vi "Local MS Auto_backup.vi"() -> ()   [LabVIEW 2016]
uses:
  Subsystems/Global Variables.vi
  <vilib>/FPGAPlugInAG/PXI-7833R/niLvFpga_Open_PXI-7833R.vi
  <vilib>/Utility/error.llb/Error Cluster From Error Code.vi
  <vilib>/rvi/errors/niLvFpgaAdjustHostInterfaceError.vi
  <vilib>/FPGAPlugInAG/PXI-7833R/niLvFpga_Reset_PXI-7833R.vi
  <vilib>/FPGAPlugInAG/PXI-7833R/niLvFpga_Close_PXI-7833R.vi
  <vilib>/rvi/interface/nirviOpenFPGA/nirviOpenFPGA.xnode
  FPGA Bitfiles/PhantomControlPI_FPGATarget_QuadCtr2_E2412E44.lvbitx
  IRISS_FPGA_IO.vi
  <vilib>/rvi/interface/nirviReadWriteControl/nirviReadWriteControl.xnode
  <vilib>/rvi/interface/nirviMethod/nirviMethod.xnode
  <vilib>/rvi/interface/nirviCloseFPGA/nirviCloseFPGA.xnode
  Library/KevinLibraryAll/labview2011/kevLib2011.lvlib
  NiFpgaLv.dll
panel:
  in  "Pause":bool caption="To M/S"
  in  "No. Cycles":u8=1
  out "Current No.":u8
  in  "L4 [deg]":dbl
  in  "L3 [mm]":dbl step=0.1
  in  "L2 [deg]":dbl
  in  "L1 [deg]":dbl
  out "Trajectory Cluster":T1
  out "Update Mdl & Traj":bool=TRUE
  out "Stage PID Cluster":T2={"Stage Z PID"={"Kp"=0.0005, "Kd"=0.001, "Ki"=0.0}, "Stage Y PID"={"Kp"=0.0003, "Kd"=0.01, "Ki"=0.0}, "Stage X PID"={"Kp"=0.0003, "Kd"=0.01, "Ki"=0.0}}
  out "L1 to L4 PID Cluster":T3={"L1 PID Gains"={"Kp"=0.005, "Kd"=0.5, "Ki"=0.0005}, "L2 PID Gains"={"Kp"=0.01, "Kd"=1.0, "Ki"=0.0005}, "L3 PID Gains"={"Kp"=0.05, "Kd"=1.0, "Ki"=0.0005}, "L4 PID Gains"={"Kp"=0.1, "Kd"=1.0, "Ki"=0.0005}}
  in  "IRISS GUI":T4(tab)
  out "X Stage out [mm] 2":dbl caption="Stage X [mm]" format="%#.4f"
  out "Z Stage out [mm] 2":dbl caption="Stage Z [mm]" format="%#.4f"
  out "Y Stage out [mm] 2":dbl caption="Stage Y [mm]" format="%#.4f"
  out "Vacuum Force [mmHg]  2":i32 caption="[mmHg]"
  out "Finished Late Counts":u16
  out "Emergency alarm":bool
  out "Remote sender engaged":bool
  in  "L2 PID Gains":cluster{"Kp":dbl, "Kd":dbl, "Ki":dbl}={"Kp"=0.01, "Kd"=1.0, "Ki"=0.005}
  in  "L3 PID Gains":cluster{"Kp":dbl, "Kd":dbl, "Ki":dbl}={"Kp"=0.05, "Kd"=1.0, "Ki"=0.0005}
  in  "L4 PID Gains":cluster{"Kp":dbl, "Kd":dbl, "Ki":dbl}={"Kp"=0.1, "Kd"=0.1, "Ki"=0.0005}
  in  "L1 PID Gains":cluster{"Kp":dbl, "Kd":dbl, "Ki":dbl}={"Kp"=0.01, "Kd"=0.5, "Ki"=0.001}
  out "Current System State":T5(ring)
  out "State changing":bool
  out "Tip out Posit":dbl[](array[numeric]) caption="Position [mm]" format="%#.3f"
  out "Tip cmd Posit":dbl[](array[numeric]) caption="Command [mm]" format="%#.3f"
  out "L4 out Posit":dbl caption="y [deg]" format="%#.2g"
  out "L4 cmd Posit":dbl caption="r [deg]" format="%#.2g"
  out "L3 out Posit":dbl caption="y [mm]" format="%#.2g"
  out "L3 cmd Posit":dbl caption="r [mm]" format="%#.2g"
  out "L2 out Posit":dbl caption="y [deg]" format="%#.2g"
  out "L2 cmd Posit":dbl caption="r [deg]" format="%#.2g"
  out "L1 out Posit":dbl caption="y [deg]" format="%#.2g"
  out "L1 cmd Posit":dbl caption="r [deg]" format="%#.2g"
  out "State Flag Array":bool[](array[boolean])
  out "Irrigation Engaged? 2":bool caption="Irrigation Engaged"
  in  "Joint Limits":dbl[][](array[numeric])=[[-8.0, 50.0], [-35.0, 35.0], [-5.0, 20.0], [-180.0, 180.0]] format="%#.3g"
  out "First Trk Pt":dbl[](array[numeric]) format="%#.3g"
  in  "Offset Home 2 RCM":dbl[](array[numeric])=[-7.7, 37.0, 55.0, 0.0] format="%#.3g"
  out "Error(s) Out on Program End":errorcluster
  out "L4 Chart":dbl(graph)
  out "L3 Chart":dbl(graph)
  out "L2 Chart":dbl(graph)
  out "L1 Chart":dbl(graph)
  in  "Clear Charts":bool
  out "AC Pressure [mmHg]":sgl
  out "Elaspsed Time":sgl
  in  "File Path":path=path "C:/KevData1.txt"
  in  "Take IOP Data":bool
  out "IOP File Exists":bool
  in  "Seconds of Data":sgl=5.0
  in  "Irrigation?":bool
  in  "PID ON/OFF":bool
  in  "Vac PID Gains":cluster{"Kp":dbl, "Kd":dbl, "Ki":dbl, "Ts":dbl}={"Kp"=5.0, "Kd"=0.0, "Ki"=5.0, "Ts"=0.01}
  in  "Vac Cmd":sgl min=0 max=100 step=1 format="%#_13g"
  in  "Target IOP":sgl=20.0 min=0 max=100 step=1 format="%#_13g"
  out "IOP Ctrl":T6(graph)
  out "Pressure Sensors":T7(graph)
  in  "Remote Control Source":u16(ring) caption="Remote Source" items=["Surgical Console", "Joystick"]
  in  "Reset Joystick":bool caption="Encoder Reset"
  in  "max limit [mmHg]":dbl=600.0
  out "OCT Z out [mm]":dbl caption="OCT Out Z [mm]" format="%#.4f"
  out "OCT Z cmd [mm]":dbl=6.0 caption="OCT Z Ref [mm]" min=0.0 max=12.0 step=0.5
  in  "OCT Z PID Gains":cluster{"Kp":dbl, "Kd":dbl, "Ki":dbl}={"Kp"=0.0003, "Kd"=0.0001, "Ki"=0.01}
  out "Z Stage out [mm]":dbl caption="Output Z [mm]" format="%#.4f"
  out "Z Stage cmd [mm]":dbl=6.0 caption="Reference Z [mm]" min=0.0 max=12.0 step=0.5
  out "Y Stage out [mm]":dbl caption="Output Y [mm]" format="%#.4f"
  out "Y Stage cmd [mm]":dbl=6.0 caption="Reference Y  [mm]" min=0.0 max=12.0 step=0.5
  out "X Stage out [mm]":dbl caption="Output X [mm]" format="%#.4f"
  out "X Stage cmd [mm]":dbl=6.0 caption="Reference X [mm]" min=0.0 max=12.0 step=0.5
  in  "Stage Z PID Gains":cluster{"Kp":dbl, "Kd":dbl, "Ki":dbl}={"Kp"=0.0005, "Kd"=0.001, "Ki"=0.0}
  in  "Stage Y PID Gains":cluster{"Kp":dbl, "Kd":dbl, "Ki":dbl}={"Kp"=0.0001, "Kd"=0.005, "Ki"=0.0}
  in  "Stage X PID Gains":cluster{"Kp":dbl, "Kd":dbl, "Ki":dbl}={"Kp"=0.0003, "Kd"=0.01, "Ki"=0.0}
  out "Irrigation Engaged?":bool
  out "Accurus Button":bool[](array[boolean]) caption="Remote Button Command"
  in  "Control: Vacuum Force":i8(slide) min=0 max=78 step=1 scale=0.0..78.0
  out "Voltage Output Ch. B":dbl(graph)
  out "Voltage Output Ch. A":dbl(graph)
  out "Accurus Engaged?":bool
  out "Vacuum Force [mmHg]":i32
  in  "Load Traj":bool caption="To M/S"
  in  "Retract":bool caption="To M/S"
  in  "Stop Accurus":bool caption="To M/S"
  in  "L3 Go Home":bool caption="To M/S"
  in  "Track":bool caption="To M/S"
  in  "Program Stop":bool
  # "Robot Status"
  # "Reserved"
  # "Tool Tip Location"
  # "L1"
  # "X\nY\nZ"
  # "X\nY\nZ"
  # "L2"
  # "Reserved"
  # "System Progress"
  # "L3"
  # "Homing finished"
  # "Reserved"
  # "M/S initialization finished"
  # "Trajecoty loading finished"
  # "Tracking initialization finished"
  # "L4"
  # "In Tracking"
  # "Notes: \n2. check state transition\n4. preview trajectory?"
  # "Vacuum"
  # "Joint Motion"
  # "Calibration"
  # "Space Deform Parameters"
  # "L1"
  # "[deg]"
  # "S"
  # "L2"
  # "[deg]"
  # "R"
  # "[deg]"
  # "L3"
  # "[mm]"
  # "T"
  # "[mm]"
  # "L4"
  # "[deg]"
  # "First Track Point"
  # "AC & PC Gap"
  # "L1"
  # "[deg]"
  # "L2"
  # "[deg]"
  # "L3"
  # "[mm]"
  # "L4"
  # "[deg]"
  # "Error Message"
  # "Tracking Joint Limits"
  # "Incision"
  # "Min."
  # "Max."
  # "L1"
  # "L1"
  # "[deg]"
  # "L2"
  # "L2"
  # "[deg]"
  # "L3"
  # "L3"
  # "[mm]"
  # "L4"
  # "L4"
  # "[deg]"
  # "Data Saving"
  # "IOP Feedback Control"
  # "XYZ Stage Control"
  # "OCT Z-Axis"
  # "Foot Pedal Buttons"
  # "Irrigation and Aspiration"
  # "Button 1"
  # "Button 2"
  # "Button 3"
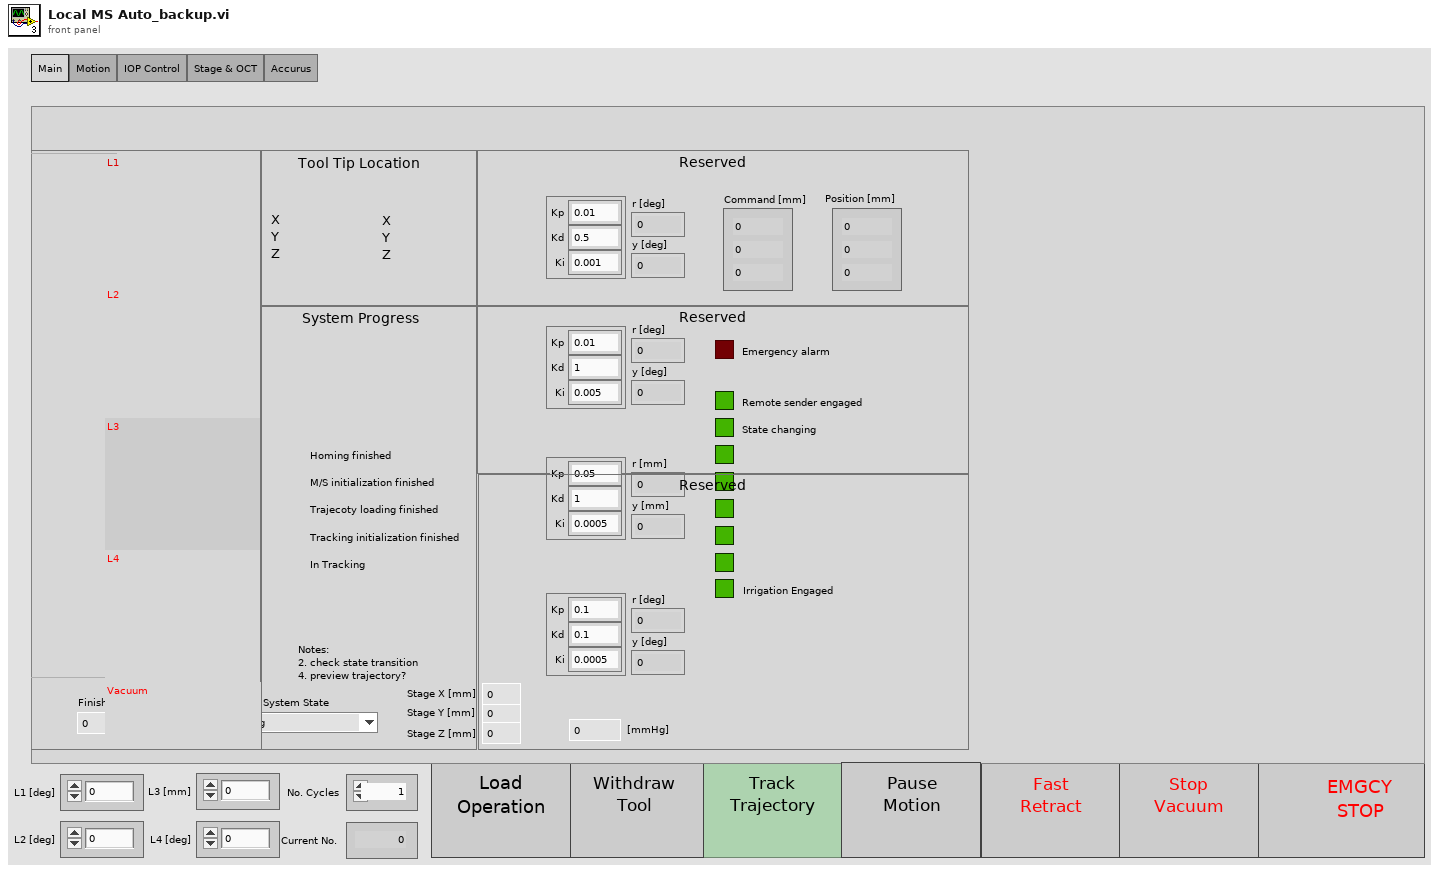
[diagram p1: front panel]
types:
  T1 = cluster{"Traj Px Array":dbl[], "Traj Py Array":dbl[], "Traj Pz Array":dbl[]}
  T2 = cluster{"Stage Z PID":cluster{"Kp":dbl, "Kd":dbl, "Ki":dbl}, "Stage Y PID":cluster{"Kp":dbl, "Kd":dbl, "Ki":dbl}, "Stage X PID":cluster{"Kp":dbl, "Kd":dbl, "Ki":dbl}}
  T3 = cluster{"L1 PID Gains":cluster{"Kp":dbl, "Kd":dbl, "Ki":dbl}, "L2 PID Gains":cluster{"Kp":dbl, "Kd":dbl, "Ki":dbl}, "L3 PID Gains":cluster{"Kp":dbl, "Kd":dbl, "Ki":dbl}, "L4 PID Gains":cluster{"Kp":dbl, "Kd":dbl, "Ki":dbl}}
  T4 = enum32{"Main", "Motion", "IOP Control", "Stage & OCT", "Accurus"}
  T5 = enum16{"Homing", "M/S Initialization", "M/S Operation", "Trajectory Loading", "Tracking Initialization", "Tracking"}
  T6 = cluster{"[0]":sgl, "[1]":sgl, "[2]":sgl, "[3]":sgl, "[4]":sgl, "[5]":sgl, "[6]":sgl, "[7]":sgl, "[8]":sgl}
  T7 = cluster{"pressure sensors[0]":sgl, "pressure sensors[1]":sgl, "pressure sensors[2]":sgl, "pressure sensors[3]":sgl, "pressure sensors[4]":sgl, "pressure sensors[5]":sgl, "pressure sensors[6]":sgl, "pressure sensors[7]":sgl, "pressure sensors[8]":sgl}
  T8 = cluster{"Prev L1 to L4 Posit":dbl[], "Prev Stage Posit":dbl[], "Prev OCT Z Posit":dbl}
  T9 = cluster{"L1 to L4 PID Cluster":cluster{"L1 PID Gains":cluster{"Kp":dbl, "Kd":dbl, "Ki":dbl}, "L2 PID Gains":cluster{"Kp":dbl, "Kd":dbl, "Ki":dbl}, "L3 PID Gains":cluster{"Kp":dbl, "Kd":dbl, "Ki":dbl}, "L4 PID Gains":cluster{"Kp":dbl, "Kd":dbl, "Ki":dbl}}, "Stage PID Cluster":cluster{"Stage Z PID":cluster{"Kp":dbl, "Kd":dbl, "Ki":dbl}, "Stage Y PID":cluster{"Kp":dbl, "Kd":dbl, "Ki":dbl}, "Stage X PID":cluster{"Kp":dbl, "Kd":dbl, "Ki":dbl}}, "OCT Z PID Gains":cluster{"Kp":dbl, "Kd":dbl, "Ki":dbl}}
  T10 = enum8{"Enabled", "Disabled", "Disabled and Grayed Out"}
  T11 = cluster{"Last L1 to L4 Posit":dbl[], "Last Stage Posit":dbl[], "Last OCT Z Posit":dbl}
  T12 = cluster{"Accurus button":bool[], "Accurus engaged?":bool, "Vacuum Force":i32, "Accurus Ch. A Vout":dbl, "Accurus Ch. B Vout":dbl, "Irrigation engaged?":bool}
  T13 = cluster{"pressure sensors[0]":sgl, "pressure sensors[1]":sgl, "pressure sensors[2]":sgl, "pressure sensors[3]":sgl, "pressure sensors[4]":sgl, "pressure sensors[5]":sgl, "pressure sensors[6]":sgl, "pressure sensors[7]":sgl, "pressure sensors[8]":sgl}[]
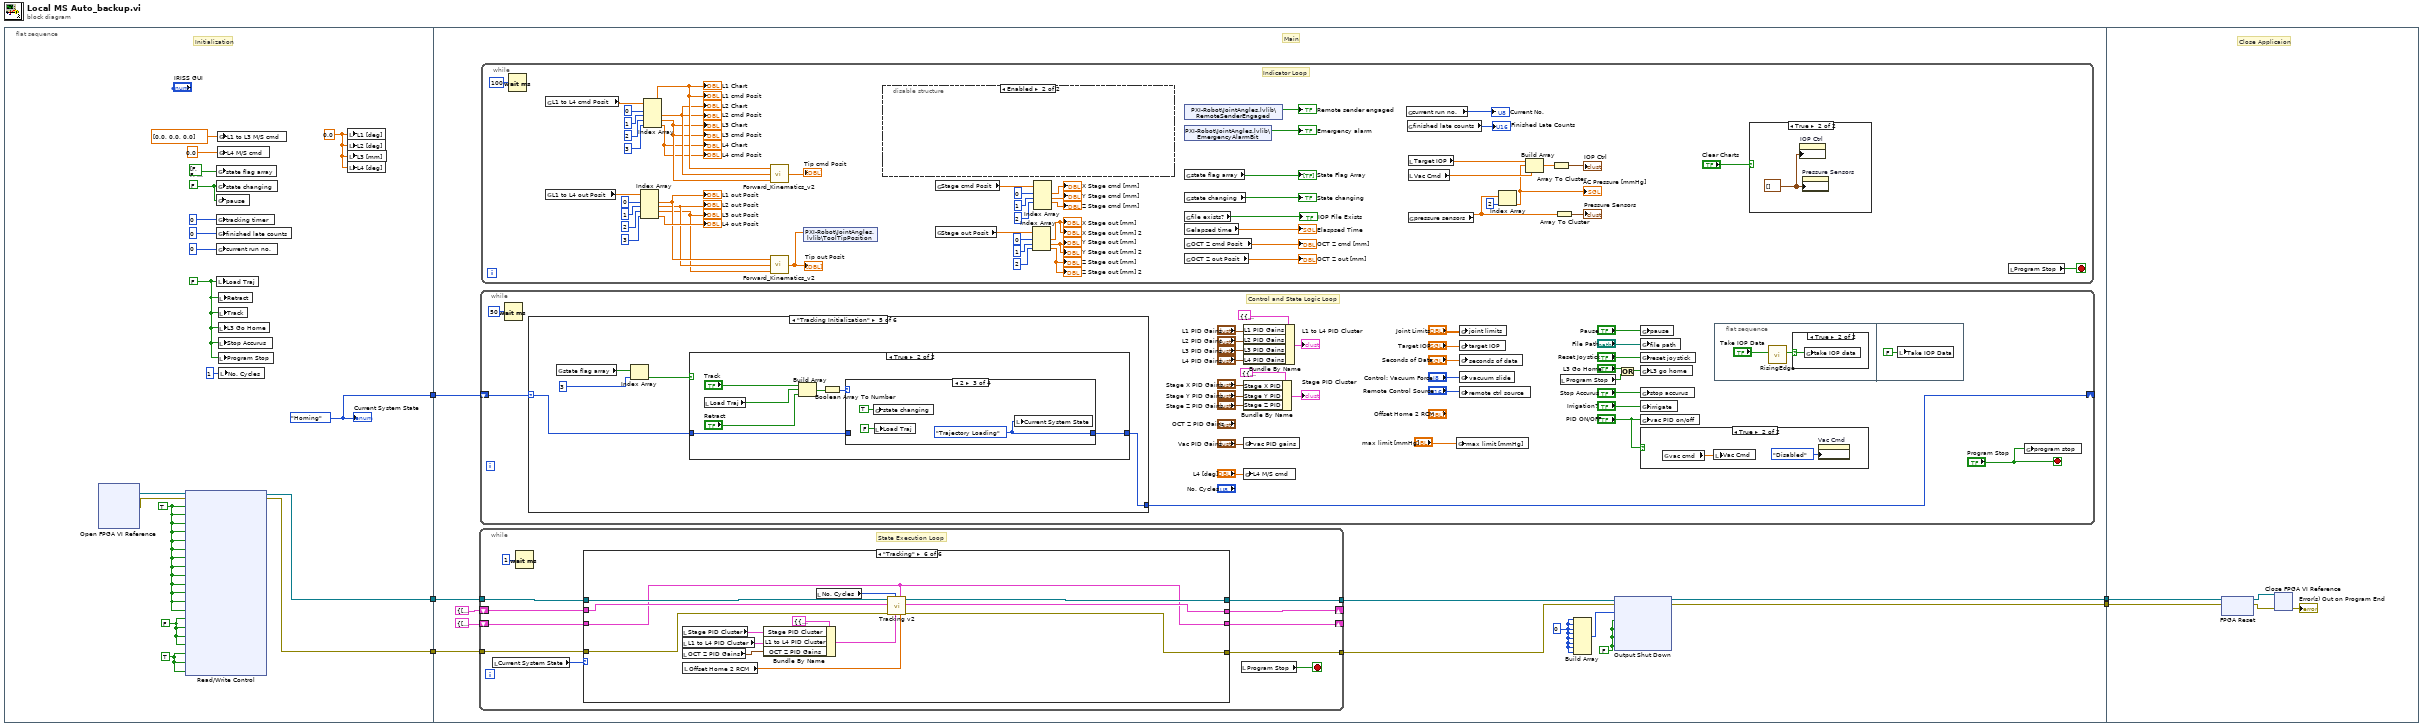
[diagram p0: block diagram]
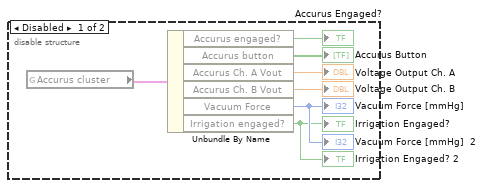
[diagram p2: hidden frame]
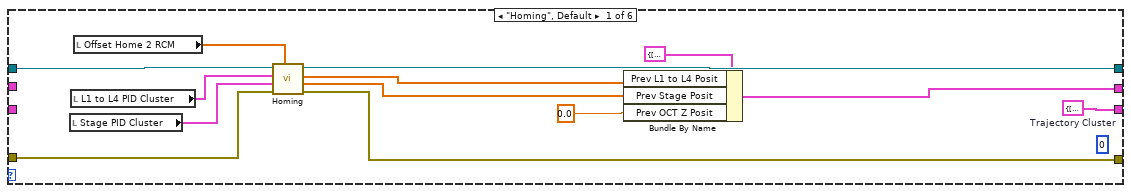
[diagram p4: hidden frame]
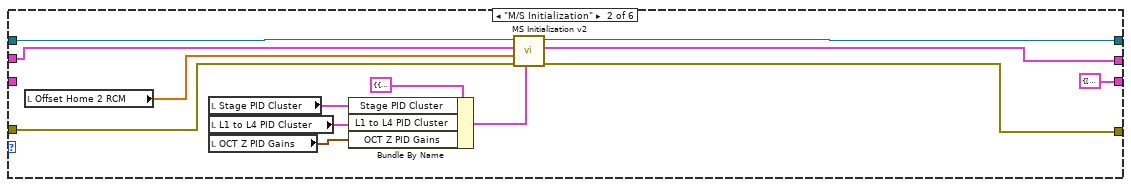
[diagram p5: hidden frame]
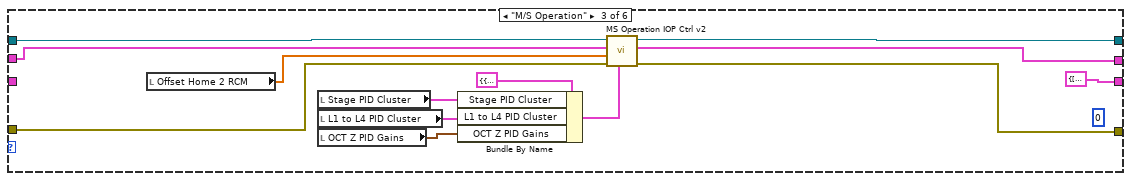
[diagram p6: hidden frame]
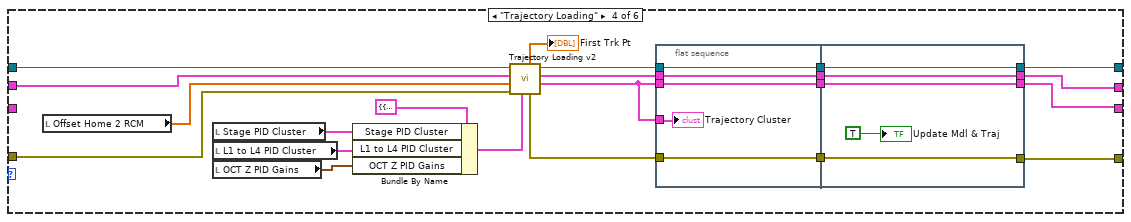
[diagram p7: hidden frame]
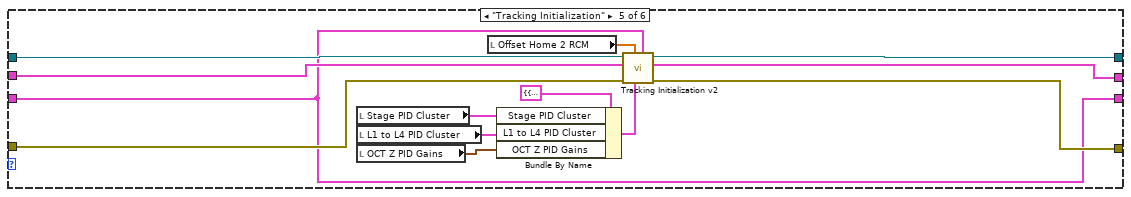
[diagram p8: hidden frame]
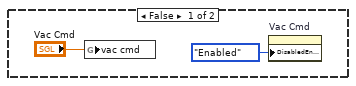
[diagram p10: hidden frame]
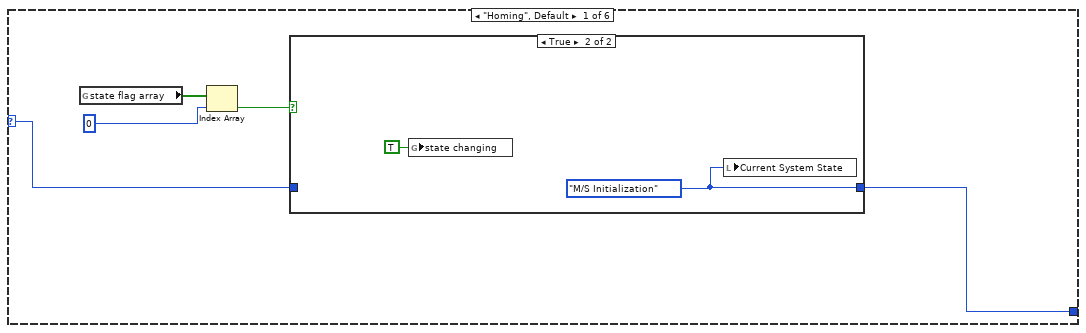
[diagram p11: hidden frame]
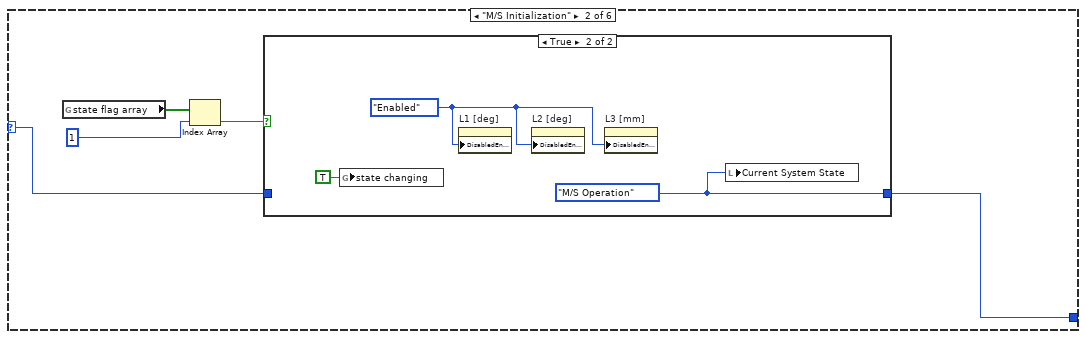
[diagram p13: hidden frame]
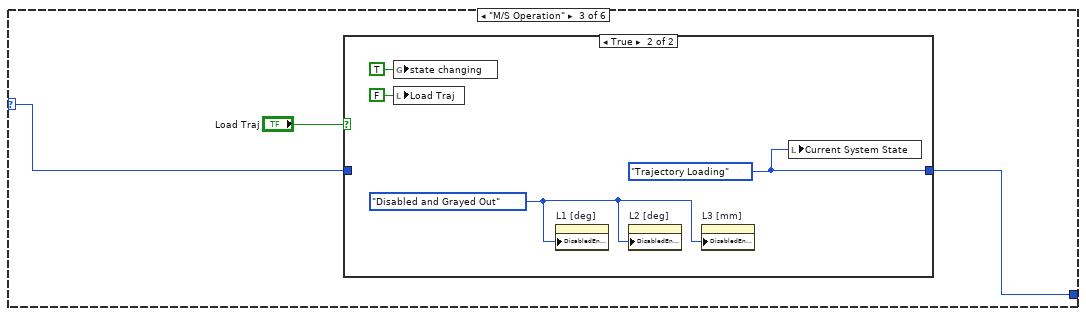
[diagram p15: hidden frame]
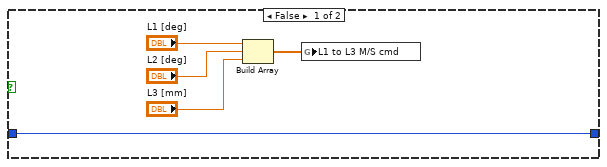
[diagram p16: hidden frame]
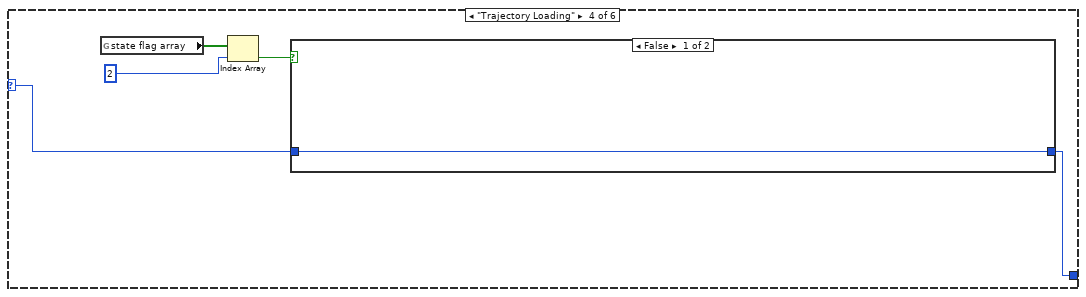
[diagram p17: hidden frame]
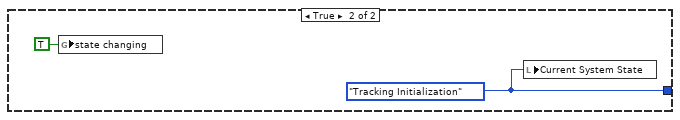
[diagram p18: hidden frame]
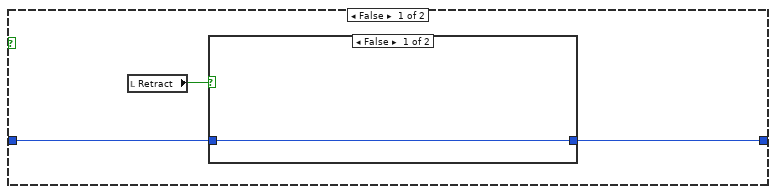
[diagram p19: hidden frame]
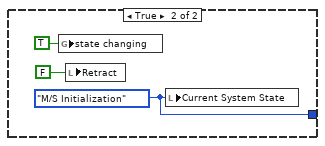
[diagram p20: hidden frame]
diagram:
  n1 = flat-sequence {
    tunnel: [w18] -> w5
    tunnel: [w17] -> w4
    tunnel: [w13] -> w3
    tunnel: w5 -> [w34]
    tunnel: w4 -> [w35]
    tunnel: w3 -> [w26]
    tunnel: [w28] -> w2
    tunnel: [w27] -> w1
    tunnel: w2 -> [w327]
    tunnel: w1 -> [w328]
    frame #0 {
      w6 = 0.0 ("L4 M/S cmd")
      w13 = T5."Homing" ("Current State")
      w14 = FALSE ("state changing")
      w22 = TRUE ("Conn0/DIO12 Button 1")
      w21 = FALSE ("Reset")
      w23 = TRUE ("Reset")
      w15 = FALSE ("program stop")
      # "Initialization"
      n2 = xnode "Open FPGA VI Reference"() -> ("FPGA VI Reference Out"=w20:refnum<k20>, "error out"=w19:errorcluster)  [unwired: 2 in]
      n3 = xnode "Read/Write Control"("FPGA VI Reference In"=w20, "error in"=w19, "Reset 1"=w23, "Reset 3"=w23, "Reset 9"=w23, "Reset 10"=w23, "Reset 11"=w23, "Reset 12"=w23, "Reset 13"=w23, "Reset 14"=w23, "Reset 15"=w23, "Reset 16"=w23, "Reset 17"=w23, "Reset C1-1"=w23, "Reset C1-4"=w23, "INHB X"=w21, "INHB Y"=w21, "INHB Z"=w21, "INHB OCT Mot"=w21, "Conn0/DIO12 Button 1"=w22, "Conn0/DIO13 Button 2"=w22, "Conn0/DIO15 Button 4"=w22) -> ("FPGA VI Reference Out"=w17:refnum<k20>, "error out"=w18:errorcluster)
      n4 = global write "Global Variables.vi" "pause"(w14) -> ()
      n5 = global write "Global Variables.vi" "state flag array"(bool[] [FALSE, FALSE, FALSE, FALSE, FALSE, FALSE, FALSE, FALSE, FALSE] ("state flag array")) -> ()
      n6 = global write "Global Variables.vi" "state changing"(w14) -> ()
      n7 = global write "Global Variables.vi" "tracking timer"(0 ("finished late counts")) -> ()
      n8 = global write "Global Variables.vi" "finished late counts"(u16 0 ("finished late counts")) -> ()
      n9 = global write "Global Variables.vi" "current run no."(u8 0 ("current run no.")) -> ()
      n10 = local write "Load Traj"(w15) -> ()
      n11 = global write "Global Variables.vi" "L1 to L3 M/S cmd"(dbl[] [0.0, 0.0, 0.0] ("L1 to L3 M/S cmd")) -> ()
      n12 = global write "Global Variables.vi" "L4 M/S cmd"(0.0 ("L4 M/S cmd")) -> ()
      n13 = local write "Retract"(w15) -> ()
      n14 = local write "Track"(w15) -> ()
      n15 = local write "L3 Go Home"(w15) -> ()
      n16 = local write "Stop Accurus"(w15) -> ()
      n17 = local write "Program Stop"(w15) -> ()
      n18 = local write "No. Cycles"(1 ("No. Cycles")) -> ()
      n19 = local write "L1 [deg]"(w6) -> ()
      n20 = local write "L2 [deg]"(w6) -> ()
      n21 = local write "L3 [mm]"(w6) -> ()
      n22 = local write "L4 [deg]"(w6) -> ()
      "Current System State" <- w13
    }
    frame #1 {
      w32 = FALSE
      w25 = i16 0 ("element")
      # "Main"
      n23 = while {
        tunnel: w35 -> [w107]
        tunnel: w34 -> [w106]
        tunnel: [w105] -> w30
        tunnel: [w104] -> w29
        shift-right: [w102] -> _
        shift-left: T8 {"Prev L1 to L4 Posit"=[0.0, 0.0, 0.0, 0.0], "Prev Stage Posit"=[6.0, 6.0, 6.0], "Prev OCT Z Posit"=0.0} ("Prev Posit Cluster") -> [w103]
        shift-right: [w100] -> _
        shift-left: T1 {"Traj Px Array"=[], "Traj Py Array"=[], "Traj Pz Array"=[]} ("Trajectory Cluster") -> [w99]
        stop <- w101 stop-if-true
        # "State Execution Loop"
        n24 = local read "Current System State"() -> (w108:T5)
        n25 = Wait (ms)(milliseconds to wait=u32 1) -> ()  [unwired: 1 out]
        n26 = case shown="\"Tracking\"" w108 {
          tunnel: w107 -> [w122 w135 w148 w170 w193 w207]
          tunnel: w106 -> [w121 w134 w147 w169 w192 w206]
          tunnel: [w120 w133 w146 w152 w191 w205] -> w105
          tunnel: [w119 w132 w145 w158 w190 w204] -> w104
          tunnel: w103 -> [_ w131 w144 w168 w188 w203]
          tunnel: [w118 w130 w143 w157 w189 w202] -> w102
          tunnel: [w110 T1 {"Traj Px Array"=[], "Traj Py Array"=[], "Traj Pz Array"=[]} ("Trajectory Cluster") T1 {"Traj Px Array"=[], "Traj Py Array"=[], "Traj Pz Array"=[]} ("Trajectory Cluster") w150 w181 w196] -> w100
          tunnel: w99 -> [_ _ _ _ w181 w196]
          frame "Homing", Default {
            w110 = T1 {"Traj Px Array"=[], "Traj Py Array"=[], "Traj Pz Array"=[]}  # Trajectory Cluster
            (unwired) 0 ("Last Index")
            n27 = local read "Stage PID Cluster"() -> (w114:T2)
            n28 = local read "L1 to L4 PID Cluster"() -> (w115:T3)
            n29 = local read "Offset Home 2 RCM"() -> (w117:dbl[])
            n30 = call "Homing.vi"("Offset Home 2 RCM"=w117, "error in"=w121, "Stage PID Cluster"=w114, "L1 to L4 PID Cluster"=w115, "FPGA VI Reference In"=w122) -> ("error out"=w119:errorcluster, "Last Stage Posit"=w111:dbl[], "Last L1 to L4 Posit"=w112:dbl[], "FPGA VI Reference Out"=w120:refnum<k20>)  [unwired: 3 in]
            n31 = Bundle By Name(cluster=T8 {"Prev L1 to L4 Posit"=[-0.5409, 0.04404050915429177, -1.917656453185038, 0.02068014705882353], "Prev Stage Posit"=[6.001471972029684, 5.996134588585126, 6.000298217087839], "Prev OCT Z Posit"=-0.0} ("Prev Posit Cluster"), "Prev L1 to L4 Posit"=w112, "Prev Stage Posit"=w111, "Prev OCT Z Posit"=0.0) -> (w118:T8)
          }
          frame "M/S Initialization" {
            n32 = local read "Offset Home 2 RCM"() -> (w124:dbl[])
            n33 = local read "Stage PID Cluster"() -> (w129:T2)
            n34 = local read "L1 to L4 PID Cluster"() -> (w128:T3)
            n35 = local read "OCT Z PID Gains"() -> (w127:cluster{"Kp":dbl, "Kd":dbl, "Ki":dbl})
            n36 = Bundle By Name(cluster=T9 {"L1 to L4 PID Cluster"={"L1 PID Gains"={"Kp"=0.005, "Kd"=0.5, "Ki"=0.0005}, "L2 PID Gains"={"Kp"=0.01, "Kd"=1.0, "Ki"=0.005}, "L3 PID Gains"={"Kp"=0.05, "Kd"=1.0, "Ki"=0.0005}, "L4 PID Gains"={"Kp"=0.1, "Kd"=0.1, "Ki"=0.0005}}, "Stage PID Cluster"={"Stage Z PID"={"Kp"=0.0005, "Kd"=0.001, "Ki"=0.0}, "Stage Y PID"={"Kp"=0.0003, "Kd"=0.01, "Ki"=0.0}, "Stage X PID"={"Kp"=0.0003, "Kd"=0.01, "Ki"=0.0}}, "OCT Z PID Gains"={"Kp"=0.0003, "Kd"=0.0001, "Ki"=0.01}} ("PID Cluster"), "Stage PID Cluster"=w129, "L1 to L4 PID Cluster"=w128, "OCT Z PID Gains"=w127) -> (w125:T9)
            n37 = call "MS Initialization v2.vi"("PID Cluster"=w125, "error in"=w134, "Offset Home 2 RCM"=w124, "Prev Posit Cluster"=w131, "FPGA VI Reference In"=w135) -> ("error out"=w132:errorcluster, "Last Posit Cluster"=w130:T11, "FPGA VI Reference Out"=w133:refnum<k20>)  [unwired: 4 in]
          }
          frame "M/S Operation" {
            (unwired) 0 ("Last Index")
            n38 = local read "Offset Home 2 RCM"() -> (w137:dbl[])
            n39 = local read "Stage PID Cluster"() -> (w142:T2)
            n40 = local read "L1 to L4 PID Cluster"() -> (w141:T3)
            n41 = local read "OCT Z PID Gains"() -> (w140:cluster{"Kp":dbl, "Kd":dbl, "Ki":dbl})
            n42 = Bundle By Name(cluster=T9 {"L1 to L4 PID Cluster"={"L1 PID Gains"={"Kp"=0.005, "Kd"=0.5, "Ki"=0.0005}, "L2 PID Gains"={"Kp"=0.01, "Kd"=1.0, "Ki"=0.005}, "L3 PID Gains"={"Kp"=0.05, "Kd"=1.0, "Ki"=0.0005}, "L4 PID Gains"={"Kp"=0.1, "Kd"=0.1, "Ki"=0.0005}}, "Stage PID Cluster"={"Stage Z PID"={"Kp"=0.0005, "Kd"=0.001, "Ki"=0.0}, "Stage Y PID"={"Kp"=0.0003, "Kd"=0.01, "Ki"=0.0}, "Stage X PID"={"Kp"=0.0003, "Kd"=0.01, "Ki"=0.0}}, "OCT Z PID Gains"={"Kp"=0.0003, "Kd"=0.0001, "Ki"=0.01}} ("PID Cluster"), "Stage PID Cluster"=w142, "L1 to L4 PID Cluster"=w141, "OCT Z PID Gains"=w140) -> (w138:T9)
            n43 = call "MS Operation IOP Ctrl v2.vi"("PID Cluster"=w138, "error in"=w147, "Offset Home 2 RCM"=w137, "Prev Posit Cluster"=w144, "FPGA VI Reference In"=w148) -> ("error out"=w145:errorcluster, "Last Posit Cluster"=w143:T11, "FPGA VI Reference Out"=w146:refnum<k20>)  [unwired: 4 in]
          }
          frame "Trajectory Loading" {
            n44 = local read "Offset Home 2 RCM"() -> (w162:dbl[])
            n45 = local read "Stage PID Cluster"() -> (w167:T2)
            n46 = local read "L1 to L4 PID Cluster"() -> (w166:T3)
            n47 = local read "OCT Z PID Gains"() -> (w165:cluster{"Kp":dbl, "Kd":dbl, "Ki":dbl})
            n48 = Bundle By Name(cluster=T9 {"L1 to L4 PID Cluster"={"L1 PID Gains"={"Kp"=0.005, "Kd"=0.5, "Ki"=0.0005}, "L2 PID Gains"={"Kp"=0.01, "Kd"=1.0, "Ki"=0.005}, "L3 PID Gains"={"Kp"=0.05, "Kd"=1.0, "Ki"=0.0005}, "L4 PID Gains"={"Kp"=0.1, "Kd"=0.1, "Ki"=0.0005}}, "Stage PID Cluster"={"Stage Z PID"={"Kp"=0.0005, "Kd"=0.001, "Ki"=0.0}, "Stage Y PID"={"Kp"=0.0003, "Kd"=0.01, "Ki"=0.0}, "Stage X PID"={"Kp"=0.0003, "Kd"=0.01, "Ki"=0.0}}, "OCT Z PID Gains"={"Kp"=0.0003, "Kd"=0.0001, "Ki"=0.01}} ("PID Cluster"), "Stage PID Cluster"=w167, "L1 to L4 PID Cluster"=w166, "OCT Z PID Gains"=w165) -> (w163:T9)
            n49 = call "Trajectory Loading v2.vi"("PID Cluster"=w163, "error in"=w169, "Offset Home 2 RCM"=w162, "Prev Posit Cluster"=w168, "FPGA VI Reference In"=w170) -> ("Trajectory Cluster"=w149:T1, "Last Posit Cluster"=w156:T11, "FPGA VI Reference Out"=w154:refnum<k20>, "error out"=w160:errorcluster, "First Trk Pt"=→"First Trk Pt":dbl[])  [unwired: 1 in, 1 out]
            n50 = flat-sequence {
              tunnel: w149 -> [w175]
              tunnel: w160 -> [w174]
              tunnel: [w174] -> w159
              tunnel: w156 -> [w173]
              tunnel: [w173] -> w155
              tunnel: w154 -> [w172]
              tunnel: [w172] -> w153
              tunnel: [w171] -> w151
              tunnel: w149 -> [w171]
              tunnel: [w179] -> w158
              tunnel: w159 -> [w179]
              tunnel: [w178] -> w157
              tunnel: w155 -> [w178]
              tunnel: w153 -> [w177]
              tunnel: [w177] -> w152
              tunnel: w151 -> [w176]
              tunnel: [w176] -> w150
              frame #0 {
                "Trajectory Cluster" <- w175
              }
              frame #1 {
                "Update Mdl & Traj" <- TRUE
              }
            }
          }
          frame "Tracking Initialization" {
            n51 = local read "Stage PID Cluster"() -> (w186:T2)
            n52 = local read "L1 to L4 PID Cluster"() -> (w185:T3)
            n53 = local read "OCT Z PID Gains"() -> (w183:cluster{"Kp":dbl, "Kd":dbl, "Ki":dbl})
            n54 = local read "Offset Home 2 RCM"() -> (w187:dbl[])
            n55 = Bundle By Name(cluster=T9 {"L1 to L4 PID Cluster"={"L1 PID Gains"={"Kp"=0.005, "Kd"=0.5, "Ki"=0.0005}, "L2 PID Gains"={"Kp"=0.01, "Kd"=1.0, "Ki"=0.005}, "L3 PID Gains"={"Kp"=0.05, "Kd"=1.0, "Ki"=0.0005}, "L4 PID Gains"={"Kp"=0.1, "Kd"=0.1, "Ki"=0.0005}}, "Stage PID Cluster"={"Stage Z PID"={"Kp"=0.0005, "Kd"=0.001, "Ki"=0.0}, "Stage Y PID"={"Kp"=0.0003, "Kd"=0.01, "Ki"=0.0}, "Stage X PID"={"Kp"=0.0003, "Kd"=0.01, "Ki"=0.0}}, "OCT Z PID Gains"={"Kp"=0.0003, "Kd"=0.0001, "Ki"=0.01}} ("PID Cluster"), "Stage PID Cluster"=w186, "L1 to L4 PID Cluster"=w185, "OCT Z PID Gains"=w183) -> (w182:T9)
            n56 = call "Tracking Initialization v2.vi"("Trajectory Cluster"=w181, "PID Cluster"=w182, "Offset Home 2 RCM"=w187, "error in"=w192, "Prev Posit Cluster"=w188, "FPGA VI Reference In"=w193) -> ("error out"=w190:errorcluster, "Last Posit Cluster"=w189:T11, "FPGA VI Reference Out"=w191:refnum<k20>)  [unwired: 3 in]
          }
          frame "Tracking" {
            n57 = local read "Stage PID Cluster"() -> (w201:T2)
            n58 = local read "L1 to L4 PID Cluster"() -> (w200:T3)
            n59 = local read "OCT Z PID Gains"() -> (w199:cluster{"Kp":dbl, "Kd":dbl, "Ki":dbl})
            n60 = local read "Offset Home 2 RCM"() -> (w195:dbl[])
            n61 = Bundle By Name(cluster=T9 {"L1 to L4 PID Cluster"={"L1 PID Gains"={"Kp"=0.005, "Kd"=0.5, "Ki"=0.0005}, "L2 PID Gains"={"Kp"=0.01, "Kd"=1.0, "Ki"=0.005}, "L3 PID Gains"={"Kp"=0.05, "Kd"=1.0, "Ki"=0.0005}, "L4 PID Gains"={"Kp"=0.1, "Kd"=0.1, "Ki"=0.0005}}, "Stage PID Cluster"={"Stage Z PID"={"Kp"=0.0005, "Kd"=0.001, "Ki"=0.0}, "Stage Y PID"={"Kp"=0.0003, "Kd"=0.01, "Ki"=0.0}, "Stage X PID"={"Kp"=0.0003, "Kd"=0.01, "Ki"=0.0}}, "OCT Z PID Gains"={"Kp"=0.0003, "Kd"=0.0001, "Ki"=0.01}} ("PID Cluster"), "Stage PID Cluster"=w201, "L1 to L4 PID Cluster"=w200, "OCT Z PID Gains"=w199) -> (w197:T9)
            n62 = local read "No. Cycles"() -> (w194:u8)
            n63 = call "Tracking v2.vi"("Offset Home 2 RCM"=w195, "Trajectory Cluster"=w196, "PID Cluster"=w197, "No. Cycles"=w194, "error in"=w206, "Prev Posit Cluster"=w203, "FPGA VI Reference In"=w207) -> ("error out"=w204:errorcluster, "Last Posit Cluster"=w202:T11, "FPGA VI Reference Out"=w205:refnum<k20>)  [unwired: 2 in]
          }
        }
        n64 = local read "Program Stop"() -> (w101:bool)
      }
      n65 = while {
        shift-right: [w218] -> _
        shift-left: w26 -> [w219]
        stop <- "Program Stop" stop-if-true
        # "Control and State Logic Loop"
        n66 = Wait (ms)(milliseconds to wait=u32 50) -> ()  [unwired: 1 out]
        n67 = case shown="\"Tracking Initialization\"" w219 {
          selector: w219 -> [w250 w256 w267 w277 w285 w314]
          tunnel: [w249 w257 w266 w278 w286 w315] -> w218
          frame "Homing", Default {
            n68 = global read "Global Variables.vi" "state flag array"() -> (w251:bool[])
            n69 = Index Array(array=w251, index=0) -> (element=w248:bool)
            n70 = case shown="True" w248 {
              tunnel: [w253 w254] -> w249
              tunnel: w250 -> [w253 _]
              frame False {
                # "homing in process"
              }
              frame True {
                w254 = T5."M/S Initialization" ("Current State")
                # "finish homing"
                n71 = global write "Global Variables.vi" "state changing"(TRUE ("state changing")) -> ()
                n72 = local write "Current System State"(w254) -> ()
              }
            }
          }
          frame "M/S Initialization" {
            n73 = global read "Global Variables.vi" "state flag array"() -> (w259:bool[])
            n74 = Index Array(array=w259, index=1) -> (element=w258:bool)
            n75 = case shown="True" w258 {
              tunnel: [w261 w263] -> w257
              tunnel: w256 -> [w261 _]
              frame False {
              }
              frame True {
                w263 = T5."M/S Operation" ("Current State")
                w262 = T10."Enabled" ("Disabled")
                n76 = global write "Global Variables.vi" "state changing"(TRUE ("state changing")) -> ()
                n77 = property on="L1 [deg]" class="DigNum (strict)"("DisabledEnum"=w262) -> ()  [unwired: 2 in, 2 out]
                n78 = property on="L2 [deg]" class="DigNum (strict)"("DisabledEnum"=w262) -> ()  [unwired: 2 in, 2 out]
                n79 = property on="L3 [mm]" class="DigNum (strict)"("DisabledEnum"=w262) -> ()  [unwired: 2 in, 2 out]
                n80 = local write "Current System State"(w263) -> ()
              }
            }
          }
          frame "M/S Operation" {
            n81 = case shown="True" "Load Traj" {
              tunnel: w267 -> [w272 _]
              tunnel: [w272 w274] -> w266
              frame False {
                n82 = Build Array("L1 [deg]", "L2 [deg]", "L3 [mm]") -> (w270:dbl[])
                n83 = global write "Global Variables.vi" "L1 to L3 M/S cmd"(w270) -> ()
              }
              frame True {
                w274 = T5."Trajectory Loading" ("Current State")
                w273 = T10."Disabled and Grayed Out" ("Disabled")
                n84 = global write "Global Variables.vi" "state changing"(TRUE ("state changing")) -> ()
                n85 = local write "Load Traj"(FALSE ("Load Traj")) -> ()
                n86 = property on="L1 [deg]" class="DigNum (strict)"("DisabledEnum"=w273) -> ()  [unwired: 2 in, 2 out]
                n87 = property on="L2 [deg]" class="DigNum (strict)"("DisabledEnum"=w273) -> ()  [unwired: 2 in, 2 out]
                n88 = property on="L3 [mm]" class="DigNum (strict)"("DisabledEnum"=w273) -> ()  [unwired: 2 in, 2 out]
                n89 = local write "Current System State"(w274) -> ()
              }
            }
          }
          frame "Trajectory Loading" {
            n90 = global read "Global Variables.vi" "state flag array"() -> (w280:bool[])
            n91 = Index Array(array=w280, index=2) -> (element=w279:bool)
            n92 = case shown="False" w279 {
              tunnel: [w282 w283] -> w278
              tunnel: w277 -> [w282 _]
              frame False {
              }
              frame True {
                w283 = T5."Tracking Initialization" ("Current State")
                n93 = global write "Global Variables.vi" "state changing"(TRUE ("state changing")) -> ()
                n94 = local write "Current System State"(w283) -> ()
              }
            }
          }
          frame "Tracking Initialization" {
            n95 = global read "Global Variables.vi" "state flag array"() -> (w288:bool[])
            n96 = Index Array(array=w288, index=3) -> (element=w287:bool)
            n97 = case shown="True" w287 {
              tunnel: [w290 w300] -> w286
              tunnel: w285 -> [w291 w299]
              frame False {
                n98 = local read "Retract"() -> (w292:bool)
                n99 = case shown="False" w292 {
                  tunnel: w291 -> [w293 _]
                  tunnel: [w293 w296] -> w290
                  frame False {
                  }
                  frame True {
                    w296 = T5."M/S Initialization" ("Current State")
                    n100 = global write "Global Variables.vi" "state changing"(TRUE ("state changing")) -> ()
                    n101 = local write "Retract"(FALSE ("Load Traj")) -> ()
                    n102 = local write "Current System State"(w296) -> ()
                  }
                }
              }
              frame True {
                n103 = local read "Load Traj"() -> (w301:bool)
                n104 = Build Array("Track", w301, "Retract") -> (w303:bool[])
                n105 = Boolean Array To Number(Boolean array=w303) -> (number=w302:u32)
                n106 = case shown="2" w302 {
                  tunnel: [w304 w305 w308 w311] -> w300
                  tunnel: w299 -> [w304 _ _ _]
                  frame 0, Default {
                  }
                  frame 1 {
                    w305 = T5."Tracking" ("Current State")
                    n107 = global write "Global Variables.vi" "state changing"(TRUE ("state changing")) -> ()
                    n108 = local write "Track"(FALSE ("Track")) -> ()
                    n109 = local write "Current System State"(w305) -> ()
                  }
                  frame 2 {
                    w308 = T5."Trajectory Loading" ("Current State")
                    n110 = global write "Global Variables.vi" "state changing"(TRUE ("state changing")) -> ()
                    n111 = local write "Load Traj"(FALSE ("Load Traj")) -> ()
                    n112 = local write "Current System State"(w308) -> ()
                  }
                  frame 4 {
                    w311 = T5."M/S Initialization" ("Current State")
                    n113 = global write "Global Variables.vi" "state changing"(TRUE ("state changing")) -> ()
                    n114 = local write "Retract"(FALSE ("Load Traj")) -> ()
                    n115 = local write "Current System State"(w311) -> ()
                  }
                }
              }
            }
          }
          frame "Tracking" {
            n116 = global read "Global Variables.vi" "state flag array"() -> (w317:bool[])
            n117 = Index Array(array=w317, index=4) -> (element=w316:bool)
            n118 = case shown="True" w316 {
              tunnel: [w319 w322] -> w315
              tunnel: w314 -> [w319 w321]
              frame False {
              }
              frame True {
                n119 = local read "Retract"() -> (w320:bool)
                n120 = case shown="True" w320 {
                  tunnel: [w323 w324] -> w322
                  tunnel: w321 -> [w323 _]
                  frame False {
                  }
                  frame True {
                    w324 = T5."M/S Initialization" ("Current State")
                    n121 = global write "Global Variables.vi" "state changing"(TRUE ("state changing")) -> ()
                    n122 = local write "Retract"(FALSE ("Load Traj")) -> ()
                    n123 = local write "Current System State"(w324) -> ()
                  }
                }
              }
            }
          }
        }
        n124 = Bundle By Name(cluster=T3 {"L1 PID Gains"={"Kp"=0.005, "Kd"=0.5, "Ki"=0.0005}, "L2 PID Gains"={"Kp"=0.01, "Kd"=1.0, "Ki"=0.0005}, "L3 PID Gains"={"Kp"=0.05, "Kd"=1.0, "Ki"=0.0005}, "L4 PID Gains"={"Kp"=0.1, "Kd"=1.0, "Ki"=0.0005}} ("L1 to L4 PID Cluster 2"), "L1 PID Gains"="L1 PID Gains", "L2 PID Gains"="L2 PID Gains", "L3 PID Gains"="L3 PID Gains", "L4 PID Gains"="L4 PID Gains") -> (→"L1 to L4 PID Cluster":T3)
        n125 = Bundle By Name(cluster=T2 {"Stage Z PID"={"Kp"=0.0005, "Kd"=0.001, "Ki"=0.0}, "Stage Y PID"={"Kp"=0.0003, "Kd"=0.01, "Ki"=0.0}, "Stage X PID"={"Kp"=0.0003, "Kd"=0.01, "Ki"=0.0}} ("Stage PID Cluster 2"), "Stage X PID"="Stage X PID Gains", "Stage Y PID"="Stage Y PID Gains", "Stage Z PID"="Stage Z PID Gains") -> (→"Stage PID Cluster":T2)
        n126 = global write "Global Variables.vi" "vac PID gains"("Vac PID Gains") -> ()
        n127 = global write "Global Variables.vi" "L4 M/S cmd"("L4 [deg]") -> ()
        n128 = global write "Global Variables.vi" "max limit [mmHg]"("max limit [mmHg]") -> ()
        n129 = global write "Global Variables.vi" "joint limits"("Joint Limits") -> ()
        n130 = global write "Global Variables.vi" "target IOP"("Target IOP") -> ()
        n131 = global write "Global Variables.vi" "seconds of data"("Seconds of Data") -> ()
        n132 = global write "Global Variables.vi" "vacuum slide"("Control: Vacuum Force") -> ()
        n133 = global write "Global Variables.vi" "remote ctrl source"("Remote Control Source") -> ()
        n134 = local read "Program Stop"() -> (w221:bool)
        n135 = Or(x="L3 Go Home", y=w221) -> (x .or. y?=w222:bool)
        n136 = global write "Global Variables.vi" "pause"("Pause") -> ()
        n137 = global write "Global Variables.vi" "file path"("File Path") -> ()
        n138 = global write "Global Variables.vi" "reset joystick"("Reset Joystick") -> ()
        n139 = global write "Global Variables.vi" "L3 go home"(w222) -> ()
        n140 = global write "Global Variables.vi" "stop accurus"("Stop Accurus") -> ()
        n141 = global write "Global Variables.vi" "irrigate"("Irrigation?") -> ()
        n142 = global write "Global Variables.vi" "vac PID on/off"("PID ON/OFF") -> ()
        n143 = case shown="True" "PID ON/OFF" {
          frame False {
            n144 = global write "Global Variables.vi" "vac cmd"("Vac Cmd") -> ()
            n145 = property on="Vac Cmd" class="DigNum (strict)"("DisabledEnum"=T10."Enabled" ("Disabled")) -> ()  [unwired: 2 in, 2 out]
          }
          frame True {
            n146 = global read "Global Variables.vi" "vac cmd"() -> (w247:sgl)
            n147 = local write "Vac Cmd"(w247) -> ()
            n148 = property on="Vac Cmd" class="DigNum (strict)"("DisabledEnum"=T10."Disabled" ("Disabled")) -> ()  [unwired: 2 in, 2 out]
          }
        }
        n149 = flat-sequence {
          frame #0 {
            n150 = call "RisingEdge.vi"("Signal In"="Take IOP Data") -> ("Rising Edge"=w240:bool)  [unwired: 10 in]
            n151 = case shown="True" w240 {
              selector: w240 -> [_ w242]
              frame False {
              }
              frame True {
                n152 = global write "Global Variables.vi" "take IOP data"(w242) -> ()
              }
            }
          }
          frame #1 {
            n153 = local write "Take IOP Data"(FALSE ("Take IOP Data")) -> ()
          }
        }
        n154 = global write "Global Variables.vi" "program stop"("Program Stop") -> ()
      }
      n155 = while {
        stop <- w71 stop-if-true
        # "Indicator Loop"
        n156 = Wait (ms)(milliseconds to wait=u32 100) -> ()  [unwired: 1 out]
        n157 = global read "Global Variables.vi" "L1 to L4 cmd Posit"() -> (w63:dbl[])
        n158 = global read "Global Variables.vi" "L1 to L4 out Posit"() -> (w66:dbl[])
        n159 = Index Array(array=w66, index #1=0 ("index"), index #2=1 ("index"), index #3=2 ("index"), index #4=3 ("index")) -> (element #1=w69:dbl, element #2=w68:dbl, element #3=w67:dbl, element #4=→"L4 out Posit":dbl)
        "L3 out Posit" <- w67
        "L2 out Posit" <- w68
        "L1 out Posit" <- w69
        n160 = Index Array(array=w63, index #1=0 ("index"), index #2=1 ("index"), index #3=2 ("index"), index #4=3 ("index")) -> (element #1=w39:dbl, element #2=w38:dbl, element #3=w37:dbl, element #4=→"L4 cmd Posit" →"L4 Chart":dbl)
        "L1 cmd Posit" <- w39
        "L3 cmd Posit" <- w37
        "L2 cmd Posit" <- w38
        "L2 Chart" <- w38
        "L1 Chart" <- w39
        "L3 Chart" <- w37
        n161 = call "Forward_Kinematics_v2.vi"("theta 3"=w37, "theta 2"=w38, "theta 1"=w39) -> ("position"=→"Tip cmd Posit":dbl[])
        n162 = call "Forward_Kinematics_v2.vi"("theta 3"=w67, "theta 2"=w68, "theta 1"=w69) -> ("position"=w58:dbl[])
        "Tip out Posit" <- w58
        n163 = shared-variable "PXI-Robot\\JointAngles.lvlib\\ToolTipPosition"(w58) -> ()  [unwired: 1 in, 1 out]
        n164 = disable-structure shown="Enabled" {
          frame Disabled {
            n165 = global read "Global Variables.vi" "Accurus cluster"() -> (w97:T12)
            n166 = Unbundle By Name(w97) -> ("Accurus engaged?"=→"Accurus Engaged?":bool, "Accurus button"=→"Accurus Button":bool[], "Accurus Ch. A Vout"=→"Voltage Output Ch. A":dbl, "Accurus Ch. B Vout"=→"Voltage Output Ch. B":dbl, "Vacuum Force"=→"Vacuum Force [mmHg]" →"Vacuum Force [mmHg]  2":i32, "Irrigation engaged?"=→"Irrigation Engaged?" →"Irrigation Engaged? 2":bool)
          }
          frame Enabled {
          }
        }
        n167 = global read "Global Variables.vi" "Stage cmd Posit"() -> (w64:dbl[])
        n168 = global read "Global Variables.vi" "Stage out Posit"() -> (w65:dbl[])
        n169 = Index Array(array=w65, index #1=0 ("index"), index #2=1 ("index"), index #3=2 ("index")) -> (element #1=→"X Stage out [mm]" →"X Stage out [mm] 2":dbl, element #2=→"Y Stage out [mm]" →"Y Stage out [mm] 2":dbl, element #3=→"Z Stage out [mm]" →"Z Stage out [mm] 2":dbl)
        n170 = Index Array(array=w64, index #1=0 ("index"), index #2=1 ("index"), index #3=2 ("index")) -> (element #1=→"X Stage cmd [mm]":dbl, element #2=→"Y Stage cmd [mm]":dbl, element #3=→"Z Stage cmd [mm]":dbl)  [unwired: 1 in, 1 out]
        n171 = shared-variable "PXI-Robot\\JointAngles.lvlib\\RemoteSenderEngaged"() -> (→"Remote sender engaged":bool)  [unwired: 1 in, 1 out]
        n172 = shared-variable "PXI-Robot\\JointAngles.lvlib\\EmergencyAlarmBit"() -> (→"Emergency alarm":bool)  [unwired: 1 in, 1 out]
        n173 = global read "Global Variables.vi" "state flag array"() -> (→"State Flag Array":bool[])
        n174 = global read "Global Variables.vi" "state changing"() -> (→"State changing":bool)
        n175 = global read "Global Variables.vi" "file exists?"() -> (→"IOP File Exists":bool)
        n176 = global read "Global Variables.vi" "elapsed time"() -> (→"Elaspsed Time":sgl)
        n177 = global read "Global Variables.vi" "OCT Z cmd Posit"() -> (→"OCT Z cmd [mm]":dbl)
        n178 = global read "Global Variables.vi" "OCT Z out Posit"() -> (→"OCT Z out [mm]":dbl)
        n179 = global read "Global Variables.vi" "current run no."() -> (→"Current No.":u8)
        n180 = global read "Global Variables.vi" "finished late counts"() -> (→"Finished Late Counts":u16)
        n181 = local read "Target IOP"() -> (w47:sgl)
        n182 = local read "Vac Cmd"() -> (w48:sgl)
        n183 = global read "Global Variables.vi" "pressure sensors"() -> (w45:sgl[])
        n184 = Index Array(array=w45, index=2) -> (element=w43:sgl)
        "AC Pressure [mmHg]" <- w43
        n185 = Build Array(w47, w43, w48) -> (w46:sgl[])
        n186 = Array To Cluster(array=w46) -> (cluster=→"IOP Ctrl":T6)
        n187 = Array To Cluster(array=w45) -> (cluster=→"Pressure Sensors":T7)
        n188 = case shown="True" "Clear Charts" {
          frame False {
          }
          frame True {
            w98 = T13 [] ("History Data")
            n189 = property on="IOP Ctrl" class="WFChart (strict)"("History Data"=w98) -> ()  [unwired: 2 in, 2 out]
            n190 = property on="Pressure Sensors" class="WFChart (strict)"("History Data"=w98) -> ()  [unwired: 2 in, 2 out]
          }
        }
        n191 = local read "Program Stop"() -> (w71:bool)
      }
      n192 = Build Array(w25, w25, w25, w25, w25, w25, w25, w25) -> (w31:i16[])
      n193 = xnode "Output Shut Down"("FPGA VI Reference In"=w30, "error in"=w29, "AO"=w31, "INHB X"=w32, "INHB Y"=w32, "INHB Z"=w32, "INHB OCT Mot"=w32) -> ("FPGA VI Reference Out"=w27:refnum<k20>, "error out"=w28:errorcluster)
    }
    frame #2 {
      # "Close Applicaion"
      n194 = xnode "FPGA Reset"("FPGA VI Reference In"=w328, "error in"=w327) -> ("FPGA VI Reference Out"=w331:refnum<k20>, "error out"=w330:errorcluster)
      n195 = xnode "Close FPGA VI Reference"("FPGA VI Reference In"=w331, "error in"=w330) -> ("error out"=→"Error(s) Out on Program End":errorcluster)
    }
  }
